vi "Rotate90(DEMO).vi"() -> ()   [LabVIEW 2011]
panel:
  out "new picture 3":picture caption="新图片"
  out "new picture 2":picture caption="新图片"
  out "new picture":picture caption="新图片"
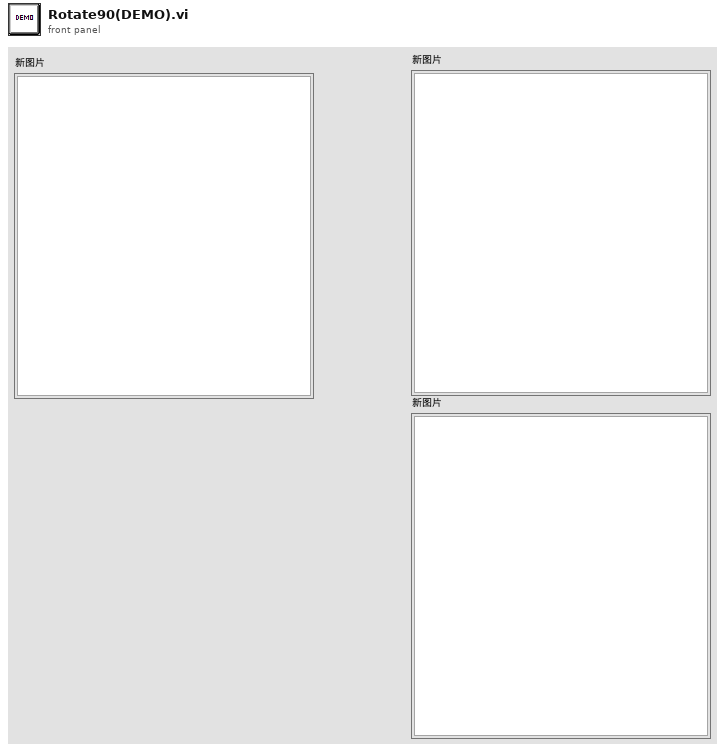
[diagram p1: front panel]
types:
  T1 = typedef "imagedata.ctl" = cluster{"image type":i32, "image depth":i32, "image":u8[], "mask":u8[], "colors":u32[], "Rectangle":cluster{"left":i16, "top":i16, "right":i16, "bottom":i16}}
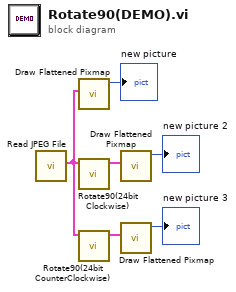
[diagram p0: block diagram]
diagram:
  n1 = call <vilib>:"Read JPEG File.vi"() -> ("image data"=w3:T1)  [unwired: 9 in, 2 out]
  n2 = call <vilib>:"Draw Flattened Pixmap.vi"("image data"=w3) -> ("new picture"=→"new picture":picture)  [unwired: 8 in]
  n3 = call "Rotate90(24bit Clockwise).vi"("image data in"=w3) -> ("image data out"=w5:T1)  [unwired: 9 in, 1 out]
  n4 = call "Rotate90(24bit CounterClockwise).vi"("image data in"=w3) -> ("image data out"=w2:T1)  [unwired: 9 in, 1 out]
  n5 = call <vilib>:"Draw Flattened Pixmap.vi"("image data"=w5) -> ("new picture"=→"new picture 2":picture)  [unwired: 8 in]
  n6 = call <vilib>:"Draw Flattened Pixmap.vi"("image data"=w2) -> ("new picture"=→"new picture 3":picture)  [unwired: 8 in]
